vi "STM Set Meta Data.vi"   [LabVIEW 2015]
doc: "Assigns the meta data cluster associated with this STM session.\n\nCopyright 2015, 2016, 2017 National Instruments Corporation\n\nLicensed under the Apache License, Version 2.0 (the \"License\"); you may not use this file except in compliance with the License.\n\n You may obtain a copy of the License at\n\n http://www.apache.org/licenses/LICENSE-2.0\n\nUnless required by applicable law or agreed to in writing, software distributed under the License is distributed on an \"AS IS\" BASIS, WITHOUT WARRANTIES OR CONDITIONS OF ANY KIND, either express or implied.\n\nSee the License for the specific language governing permissions and limitations under the License."
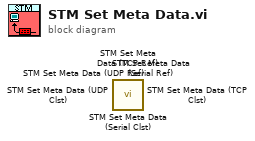
[diagram p0: block diagram]
diagram:
  n1 = call <vilib>:"STM Set Meta Data (Serial Clst).vi"() -> ()  [unwired: 10 in, 2 out]
  n2 = call <vilib>:"STM Set Meta Data (Serial Ref).vi"() -> ()  [unwired: 10 in, 2 out]
  n3 = call <vilib>:"STM Set Meta Data (UDP Clst).vi"() -> ()  [unwired: 10 in, 2 out]
  n4 = call <vilib>:"STM Set Meta Data (TCP Clst).vi"() -> ()  [unwired: 10 in, 2 out]
  n5 = call <vilib>:"STM Set Meta Data (UDP Ref).vi"() -> ()  [unwired: 10 in, 2 out]
  n6 = call <vilib>:"STM Set Meta Data (TCP Ref).vi"() -> ()  [unwired: 10 in, 2 out]
